vi "StepGeneral.vi"(0 "StepNr":i32=1, 2 "seq in":T3, 5 "Nazwa":string="Krok1") -> (13 "seq out":T2)   [LabVIEW 2020]
uses:
  controls/Data.ctl
  Global.vi
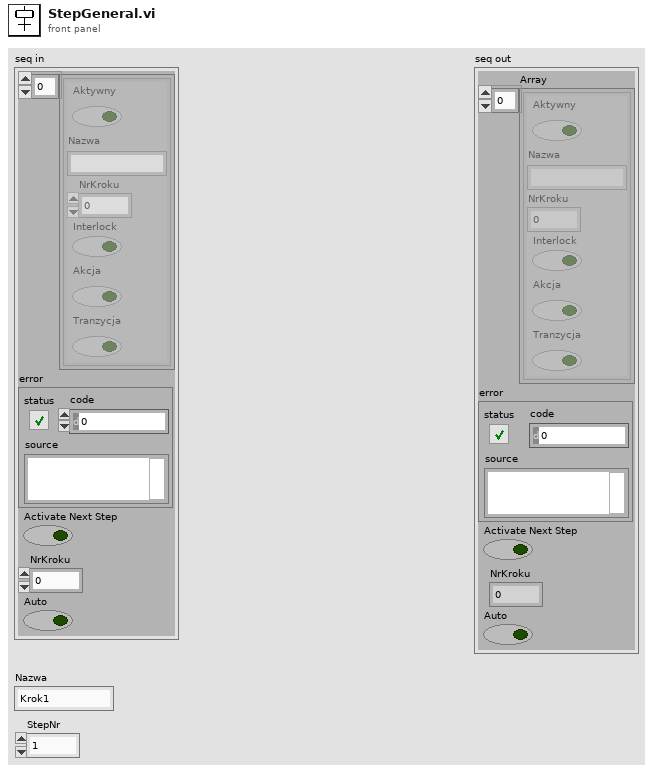
[diagram p1: front panel]
types:
  T1 = typedef "Data.ctl" = cluster{"Aktywny":bool, "Nazwa":string, "NrKroku":dbl, "Interlock":bool, "Akcja":bool, "Tranzycja":bool}
  T2 = cluster{"Array":T1[], "error":errorcluster, "Activate Next Step":bool, "NrKroku":dbl, "Auto":bool}
  T3 = cluster{T1[], "error":errorcluster, "Activate Next Step":bool, "NrKroku":dbl, "Auto":bool}
  T4 = cluster{string, "Interlock":bool, "Aktywny":bool}
  T5 = cluster{T1[], "error":errorcluster, bool, dbl, "W cyklu":bool}
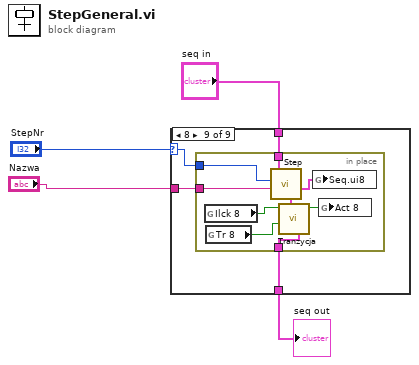
[diagram p0: block diagram]
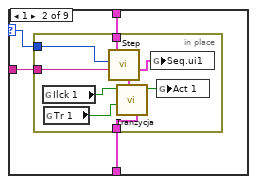
[diagram p3: hidden frame]
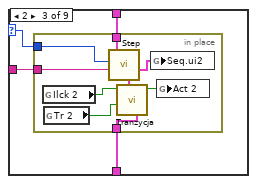
[diagram p4: hidden frame]
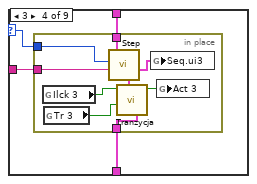
[diagram p5: hidden frame]
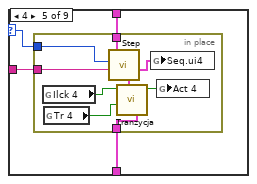
[diagram p6: hidden frame]
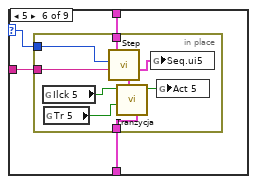
[diagram p7: hidden frame]
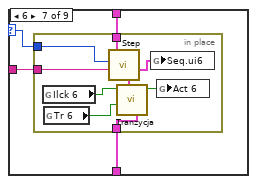
[diagram p8: hidden frame]
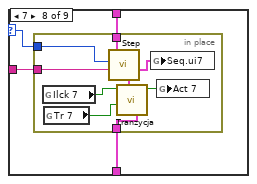
[diagram p9: hidden frame]
diagram:
  n1 = case shown="8" "StepNr" {
    selector: "StepNr" -> [_ w6 w19 w32 w45 w58 w71 w84 w97]
    tunnel: [w5 w9 w22 w35 w48 w61 w74 w87 w100] -> w1
    tunnel: "seq in" -> [w5 w8 w21 w34 w47 w60 w73 w86 w99]
    tunnel: "Nazwa" -> [_ w7 w20 w33 w46 w59 w72 w85 w98]
    frame 0, Default {
    }
    frame 1 {
      n2 = in-place {
        in-place-border: w8 -> [w17]
        in-place-border: [w16] -> w9
        in-place-border: w6 -> [w11]
        in-place-border: w7 -> [w10]
        n3 = global read "Global.vi" "Ilck 1"() -> (w14:bool)
        n4 = global read "Global.vi" "Tr 1"() -> (w12:bool)
        n5 = call "Step.vi"("input"=w17, "Nazwa"=w10, "Numeric"=w11) -> (1:w13:T4, "output cluster"=w18:T5)  [unwired: 7 in]
        n6 = call "Tranzycja.vi"("input"=w18, "Tranzycja"=w12, "Interlock"=w14) -> ("Akcja"=w15:bool, "output"=w16:T2)  [unwired: 7 in]
        n7 = global write "Global.vi" "Seq.ui1"(w13) -> ()
        n8 = global write "Global.vi" "Act 1"(w15) -> ()
      }
    }
    frame 2 {
      n9 = in-place {
        in-place-border: w21 -> [w30]
        in-place-border: [w29] -> w22
        in-place-border: w19 -> [w24]
        in-place-border: w20 -> [w23]
        n10 = global read "Global.vi" "Ilck 2"() -> (w27:bool)
        n11 = global read "Global.vi" "Tr 2"() -> (w25:bool)
        n12 = call "Step.vi"("input"=w30, "Nazwa"=w23, "Numeric"=w24) -> (1:w26:T4, "output cluster"=w31:T5)  [unwired: 7 in]
        n13 = call "Tranzycja.vi"("input"=w31, "Tranzycja"=w25, "Interlock"=w27) -> ("Akcja"=w28:bool, "output"=w29:T2)  [unwired: 7 in]
        n14 = global write "Global.vi" "Seq.ui2"(w26) -> ()
        n15 = global write "Global.vi" "Act 2"(w28) -> ()
      }
    }
    frame 3 {
      n16 = in-place {
        in-place-border: w34 -> [w43]
        in-place-border: [w42] -> w35
        in-place-border: w32 -> [w37]
        in-place-border: w33 -> [w36]
        n17 = global read "Global.vi" "Ilck 3"() -> (w40:bool)
        n18 = global read "Global.vi" "Tr 3"() -> (w38:bool)
        n19 = call "Step.vi"("input"=w43, "Nazwa"=w36, "Numeric"=w37) -> (1:w39:T4, "output cluster"=w44:T5)  [unwired: 7 in]
        n20 = call "Tranzycja.vi"("input"=w44, "Tranzycja"=w38, "Interlock"=w40) -> ("Akcja"=w41:bool, "output"=w42:T2)  [unwired: 7 in]
        n21 = global write "Global.vi" "Seq.ui3"(w39) -> ()
        n22 = global write "Global.vi" "Act 3"(w41) -> ()
      }
    }
    frame 4 {
      n23 = in-place {
        in-place-border: w47 -> [w56]
        in-place-border: [w55] -> w48
        in-place-border: w45 -> [w50]
        in-place-border: w46 -> [w49]
        n24 = global read "Global.vi" "Ilck 4"() -> (w53:bool)
        n25 = global read "Global.vi" "Tr 4"() -> (w51:bool)
        n26 = call "Step.vi"("input"=w56, "Nazwa"=w49, "Numeric"=w50) -> (1:w52:T4, "output cluster"=w57:T5)  [unwired: 7 in]
        n27 = call "Tranzycja.vi"("input"=w57, "Tranzycja"=w51, "Interlock"=w53) -> ("Akcja"=w54:bool, "output"=w55:T2)  [unwired: 7 in]
        n28 = global write "Global.vi" "Seq.ui4"(w52) -> ()
        n29 = global write "Global.vi" "Act 4"(w54) -> ()
      }
    }
    frame 5 {
      n30 = in-place {
        in-place-border: w60 -> [w69]
        in-place-border: [w68] -> w61
        in-place-border: w58 -> [w63]
        in-place-border: w59 -> [w62]
        n31 = global read "Global.vi" "Ilck 5"() -> (w66:bool)
        n32 = global read "Global.vi" "Tr 5"() -> (w64:bool)
        n33 = call "Step.vi"("input"=w69, "Nazwa"=w62, "Numeric"=w63) -> (1:w65:T4, "output cluster"=w70:T5)  [unwired: 7 in]
        n34 = call "Tranzycja.vi"("input"=w70, "Tranzycja"=w64, "Interlock"=w66) -> ("Akcja"=w67:bool, "output"=w68:T2)  [unwired: 7 in]
        n35 = global write "Global.vi" "Seq.ui5"(w65) -> ()
        n36 = global write "Global.vi" "Act 5"(w67) -> ()
      }
    }
    frame 6 {
      n37 = in-place {
        in-place-border: w73 -> [w82]
        in-place-border: [w81] -> w74
        in-place-border: w71 -> [w76]
        in-place-border: w72 -> [w75]
        n38 = global read "Global.vi" "Ilck 6"() -> (w79:bool)
        n39 = global read "Global.vi" "Tr 6"() -> (w77:bool)
        n40 = call "Step.vi"("input"=w82, "Nazwa"=w75, "Numeric"=w76) -> (1:w78:T4, "output cluster"=w83:T5)  [unwired: 7 in]
        n41 = call "Tranzycja.vi"("input"=w83, "Tranzycja"=w77, "Interlock"=w79) -> ("Akcja"=w80:bool, "output"=w81:T2)  [unwired: 7 in]
        n42 = global write "Global.vi" "Seq.ui6"(w78) -> ()
        n43 = global write "Global.vi" "Act 6"(w80) -> ()
      }
    }
    frame 7 {
      n44 = in-place {
        in-place-border: w86 -> [w95]
        in-place-border: [w94] -> w87
        in-place-border: w84 -> [w89]
        in-place-border: w85 -> [w88]
        n45 = global read "Global.vi" "Ilck 7"() -> (w92:bool)
        n46 = global read "Global.vi" "Tr 7"() -> (w90:bool)
        n47 = call "Step.vi"("input"=w95, "Nazwa"=w88, "Numeric"=w89) -> (1:w91:T4, "output cluster"=w96:T5)  [unwired: 7 in]
        n48 = call "Tranzycja.vi"("input"=w96, "Tranzycja"=w90, "Interlock"=w92) -> ("Akcja"=w93:bool, "output"=w94:T2)  [unwired: 7 in]
        n49 = global write "Global.vi" "Seq.ui7"(w91) -> ()
        n50 = global write "Global.vi" "Act 7"(w93) -> ()
      }
    }
    frame 8 {
      n51 = in-place {
        in-place-border: w99 -> [w108]
        in-place-border: [w107] -> w100
        in-place-border: w97 -> [w102]
        in-place-border: w98 -> [w101]
        n52 = global read "Global.vi" "Ilck 8"() -> (w105:bool)
        n53 = global read "Global.vi" "Tr 8"() -> (w103:bool)
        n54 = call "Step.vi"("input"=w108, "Nazwa"=w101, "Numeric"=w102) -> (1:w104:T4, "output cluster"=w109:T5)  [unwired: 7 in]
        n55 = call "Tranzycja.vi"("input"=w109, "Tranzycja"=w103, "Interlock"=w105) -> ("Akcja"=w106:bool, "output"=w107:T2)  [unwired: 7 in]
        n56 = global write "Global.vi" "Seq.ui8"(w104) -> ()
        n57 = global write "Global.vi" "Act 8"(w106) -> ()
      }
    }
  }
  "seq out" <- w1
